vi "Steve_Tan_UV_Histogram.vi"() -> (5 "Plug in titles":string[](array[string]), 7 "Plug in values":string[](array[string]))   [LabVIEW 2010]
uses:
  Globals/Plug_in_data_global.vi
  Globals/Meas_global.vi
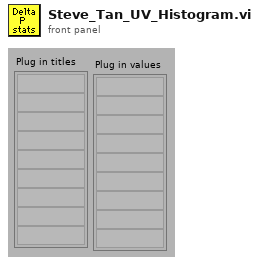
[diagram p1: front panel]
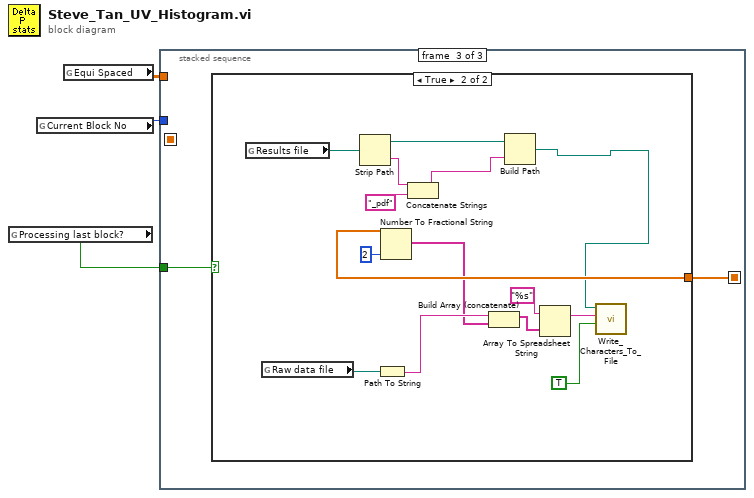
[diagram p0: block diagram]
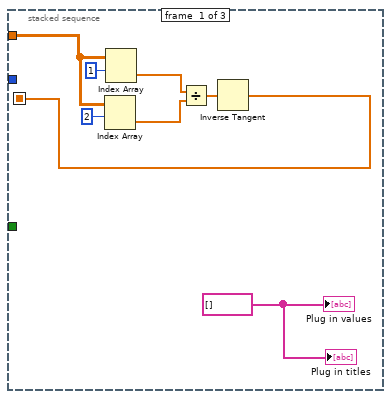
[diagram p2: hidden frame]
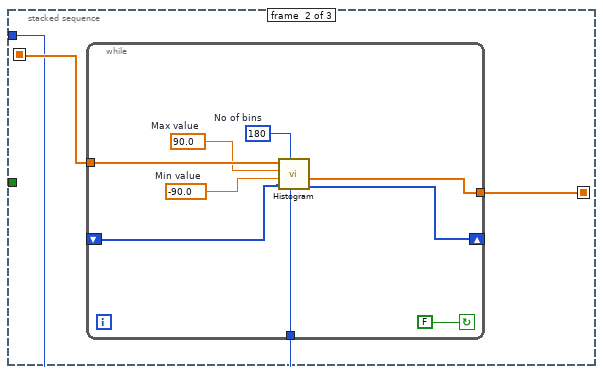
[diagram p3: hidden frame]
diagram:
  n1 = global read "Meas_global.vi" "Processing last block?"() -> (w1:bool)
  n2 = global read "Meas_global.vi" "Current Block No"() -> (w2:i32)
  n3 = global read "Plug_in_data_global.vi" "Equi Spaced"() -> (w3:dbl[][])
  n4 = stacked-sequence {
    seq-local: [w5 _ _] -> [_ w14 _]
    seq-local: [_ w13 _] -> [_ _ w24]
    tunnel: w3 -> [w10 _ _]
    tunnel: w2 -> [_ w12 _]
    tunnel: w1 -> [_ _ w25]
    frame #0 {
      w4 = string[] [] ("Plug in values")
      n5 = Index Array(array=w10, index (row)=2) -> (element=w7:dbl[])  [unwired: 1 in]
      n6 = Index Array(array=w10, index (row)=1) -> (element=w6:dbl[])  [unwired: 1 in]
      n7 = Divide(x=w6, y=w7) -> (x/y=w8:dbl[])
      n8 = Inverse Tangent(1:w8) -> (0:w5:dbl[])
      "Plug in values" <- w4
      "Plug in titles" <- w4
    }
    frame #1 {
      n9 = while {
        tunnel: w12 -> [w17]
        tunnel: [w18] -> w13
        shift-left: _ -> [w16]
        shift-right: [w21] -> _
        tunnel: w14 -> [w22]
        stop <- FALSE continue-if-true
        w19 = 90.0  # Max value
        w20 = -90.0  # Min value
        w23 = 180  # No of bins
        n10 = call "Histogram.vi"("Current Block No"=w17, "No of bins"=w23, "Shift Hist"=w16, "Min value"=w20, "Max value"=w19, "X"=w22) -> ("Shift Hist"=w21:i32[], "Histogram of X"=w18:dbl[])  [unwired: 2 in, 1 out]
      }
    }
    frame #2 {
      n11 = case shown="True" w25 {
        tunnel: w24 -> [_ w40]
        frame False {
        }
        frame True {
          n12 = global read "Meas_global.vi" "Results file"() -> (w27:path)
          n13 = global read "Meas_global.vi" "Raw data file"() -> (w28:path)
          n14 = Strip Path(path=w27) -> (stripped path=w33:path, name=w30:string)
          n15 = Path To String(path=w28) -> (string=w38:string)
          n16 = Number To Fractional String(number=w40, precision (6)=i16 2) -> (F-format string=w37:string[])  [unwired: 2 in]
          n17 = Concatenate Strings(w30, "_pdf" ("Substring")) -> (w32:string)
          n18 = Build Array (concatenate)(w38, w37) -> (w36:string[])
          n19 = Build Path(base path=w33, name or relative path=w32) -> (appended path=w26:path)
          n20 = Array To Spreadsheet String(array=w36, 3:"%s" ("format string")) -> (spreadsheet string=w35:string)  [unwired: 1 in]
          n21 = call "Write_Characters_To_File.vi"("file path (dialog if empty)"=w26, "character string"=w35, "append to file? (new file:F)"=TRUE) -> ()  [unwired: 5 in, 1 out]
        }
      }
    }
  }
